vi "Set Debounce Period.vi"(8 "error in (no error)":errorcluster, 10 "debounce (100)":u32=100, 11 "Template in":refnum<class "Template.lvclass">) -> (0 "error out":errorcluster, 3 "Template out":refnum<class "Template.lvclass">)   [LabVIEW 2011, in "Tinkerforge.lvlib" / "Template.lvclass"]
doc: "This VI sets the debounce period of the callbacks. This period is used if the threshold configuration leads to initial triggering of the callback."
uses:
  Template.lvclass
  Device/Device.lvclass
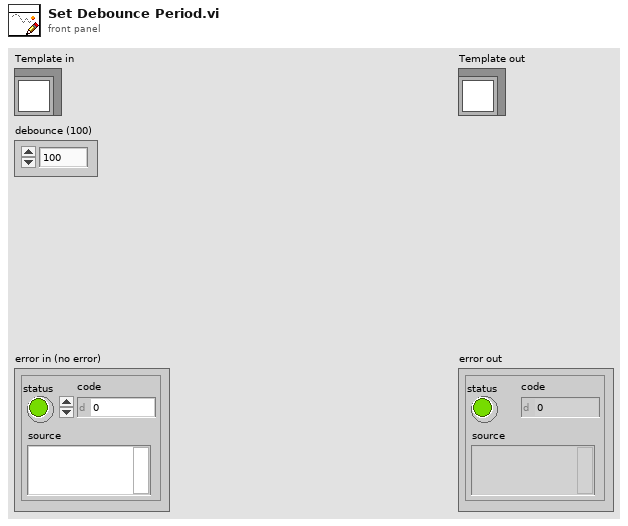
[diagram p1: front panel]
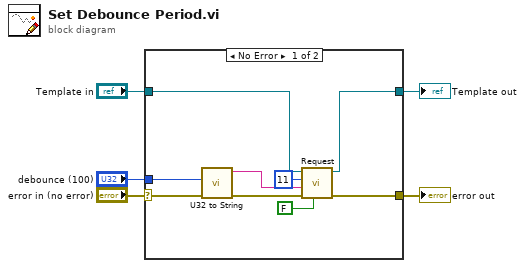
[diagram p0: block diagram]
diagram:
  n1 = case shown="No Error" "error in (no error)" {
    selector: "error in (no error)" -> [w9 w16]
    tunnel: [w10 w16] -> w4
    tunnel: [w13 w15] -> w2
    tunnel: "Template in" -> [w14 w15]
    tunnel: "debounce (100)" -> [w7 _]
    frame No Error {
      n2 = call "U32 to String.vi"("Error In"=w9, "U32"=w7) -> ("Error Out"=w8:errorcluster, "String out"=w6:string)  [unwired: 8 in]
      n3 = call "Request.vi"("Response"=FALSE, "error in (no error)"=w8, "Data"=w6, "Function ID"=u8 11, "Device in"=w14) -> ("error out"=w10:errorcluster, "Device out"=w13:refnum<class "Template.lvclass">)  [unwired: 2 in, 3 out]
    }
    frame Error {
    }
  }
  "error out" <- w4
  "Template out" <- w2
